vi "Conceptual Patterns.vi"() -> ()   [LabVIEW 2015]
panel:
  out "Array 11":bool[][](array[boolean])=[[TRUE, TRUE, TRUE], [TRUE, TRUE, TRUE], [TRUE, TRUE, TRUE]]
  out "Array 10":bool[][](array[boolean])=[[FALSE, FALSE, TRUE, TRUE, TRUE, FALSE, FALSE], [TRUE, TRUE, FALSE, TRUE, FALSE, TRUE, TRUE], [TRUE, FALSE, FALSE, FALSE, FALSE, FALSE, TRUE], [TRUE, TRUE, FALSE, FALSE, FALSE, TRUE, TRUE], [TRUE, FALSE, FALSE, FALSE, FALSE, FALSE, TRUE], [TRUE, TRUE, FALSE, TRUE, FALSE, TRUE, TRUE], [FALSE, FALSE, TRUE, TRUE, TRUE, FALSE, FALSE]]
  out "Array 9":bool[][](array[boolean])=[[FALSE, FALSE, TRUE, TRUE, TRUE, FALSE, FALSE], [TRUE, TRUE, FALSE, TRUE, FALSE, TRUE, TRUE], [TRUE, FALSE, FALSE, FALSE, FALSE, FALSE, TRUE], [TRUE, TRUE, FALSE, FALSE, FALSE, TRUE, TRUE], [TRUE, FALSE, FALSE, FALSE, FALSE, FALSE, TRUE], [TRUE, TRUE, FALSE, TRUE, FALSE, TRUE, TRUE], [FALSE, FALSE, TRUE, TRUE, TRUE, FALSE, FALSE]]
  out "Array 8":bool[][](array[boolean])=[[FALSE, FALSE, TRUE, FALSE, TRUE, FALSE, FALSE], [TRUE, FALSE, FALSE, TRUE, FALSE, FALSE, TRUE], [FALSE, TRUE, TRUE, TRUE, TRUE, TRUE, FALSE], [TRUE, FALSE, TRUE, FALSE, TRUE, FALSE, TRUE], [FALSE, TRUE, TRUE, TRUE, TRUE, TRUE, FALSE], [TRUE, FALSE, FALSE, TRUE, FALSE, FALSE, TRUE], [FALSE, FALSE, TRUE, FALSE, TRUE, FALSE, FALSE]]
  out "Array 7":bool[][](array[boolean])=[[FALSE, FALSE, FALSE, TRUE, FALSE, FALSE, FALSE], [TRUE, TRUE, FALSE, TRUE, FALSE, TRUE, TRUE], [TRUE, TRUE, FALSE, FALSE, FALSE, TRUE, TRUE], [TRUE, TRUE, FALSE, FALSE, FALSE, TRUE, TRUE], [TRUE, TRUE, FALSE, FALSE, FALSE, TRUE, TRUE], [TRUE, TRUE, FALSE, TRUE, FALSE, TRUE, TRUE], [FALSE, FALSE, FALSE, TRUE, FALSE, FALSE, FALSE]]
  out "Array 6":bool[][](array[boolean])=[[TRUE, TRUE, TRUE, TRUE, TRUE], [TRUE, TRUE, TRUE, TRUE, TRUE], [TRUE, TRUE, FALSE, TRUE, TRUE], [TRUE, TRUE, TRUE, TRUE, TRUE], [TRUE, TRUE, TRUE, TRUE, TRUE]]
  out "Array 5":bool[][](array[boolean])=[[TRUE, TRUE, TRUE, TRUE], [TRUE, FALSE, FALSE, TRUE], [TRUE, TRUE, TRUE, TRUE]]
  out "Array 4":bool[][](array[boolean])=[[TRUE, TRUE, TRUE, TRUE], [FALSE, FALSE, FALSE, FALSE], [TRUE, TRUE, TRUE, TRUE]]
  out "Array 3":bool[][](array[boolean])=[[TRUE, TRUE, TRUE, TRUE], [FALSE, FALSE, FALSE, FALSE], [TRUE, TRUE, TRUE, TRUE]]
  out "Array 2":bool[][](array[boolean])=[[TRUE, TRUE, TRUE, TRUE], [TRUE, TRUE, TRUE, TRUE]]
  out "Array":bool[][](array[boolean])=[[TRUE, TRUE], [TRUE, TRUE]]
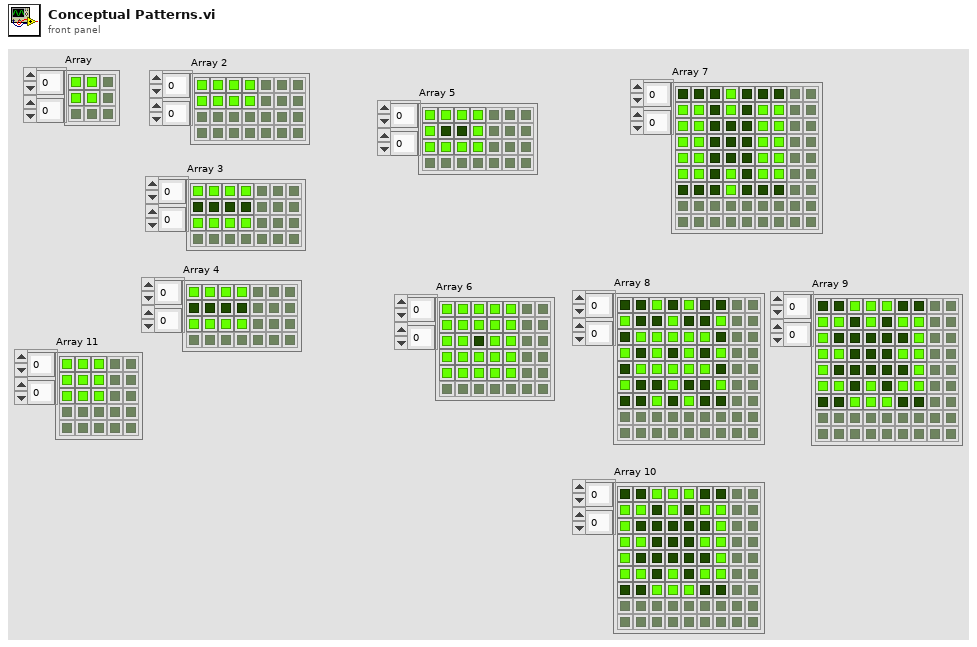
[diagram p1: front panel]
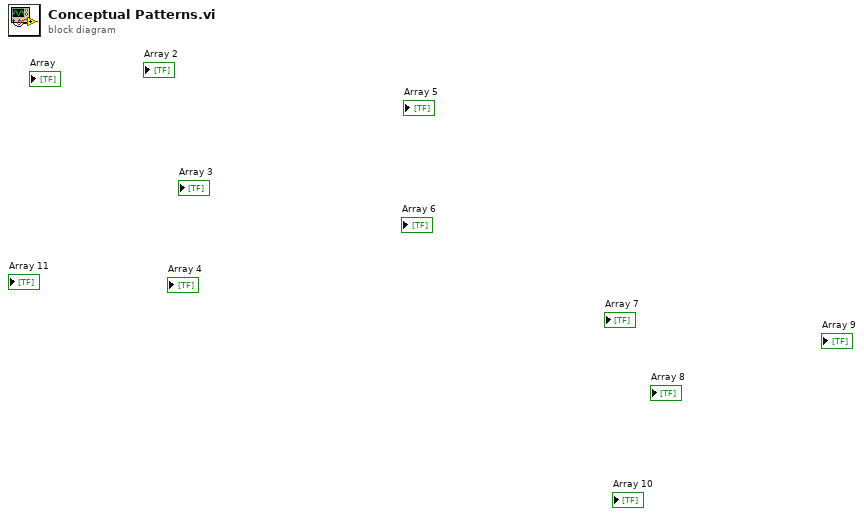
[diagram p0: block diagram]
diagram:
